vi "h.ACQ.StreamSpectraAllChannels.vi"(6 "power scales and offsets":i32[][](array[numeric]), 8 "error in":errorcluster, 11 "Connection ID":refnum<k5>) -> (0 "error out":errorcluster, 2 "Spectral Data":T1 {"Spectrum"."Spectrum, db" format="%_8g"}, 3 "Connection ID out":refnum<k5>)   [LabVIEW 2016, in "h.Library.lvlib"]
uses:
  h.Library.lvlib
  COMM/CTL/h.COMM.Command Status Enum.ctl
  COMM/CTL/h.COMM.RequestCommandOptions.ctl
  CTL/h.ACQ.SpectralData.ctl
  CTL/h.ACQ.Spectrum.ctl
panel:
  out "Message Length":u16
  out "Request Option Echo":T3=enum."Suppress Message"
  out "Message":string
  out "Content":u8[](array[numeric])
  out "Content Length":u32
  out "Status":T4
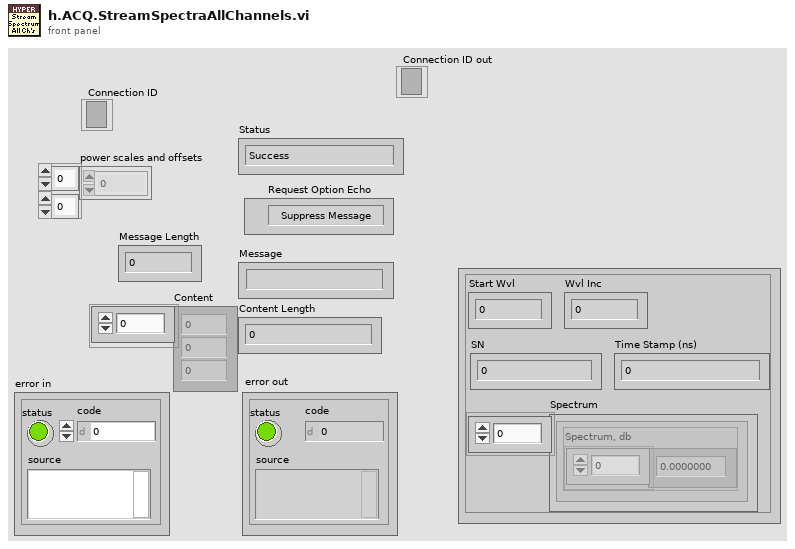
[diagram p1: front panel]
types:
  T1 = typedef "h.Library.lvlib/h.ACQ.SpectralData.ctl" = cluster{"Spectrum":T2[], "Start Wvl":dbl, "Wvl Inc":dbl, "SN":u64, "Time Stamp (ns)":u64}
  T2 = typedef "h.Library.lvlib/h.ACQ.Spectrum.ctl" = cluster{"Spectrum, db":dbl[]}
  T3 = typedef "h.Library.lvlib/h.COMM.RequestCommandOptions.ctl" = enum8{"None", "Suppress Message", "Suppress Content", "Compress"}
  T4 = typedef "h.Library.lvlib/h.COMM.Command Status Enum.ctl" = enum8{"Success", "Failed", "Error", "AccessDenied", "InvalidCommand", "InvalidNumberArguments", "InvalidArgument", ""}
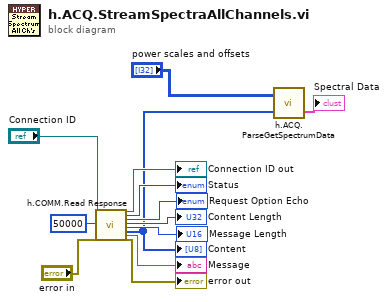
[diagram p0: block diagram]
diagram:
  n1 = call "h.COMM.Read Response.vi"("Connection ID"="Connection ID", "Timeout"=50000, "error in"="error in") -> ("Connection ID"=→"Connection ID out":refnum<k5>, "Status"=→"Status":T4, "Request Option Echo"=→"Request Option Echo":T3, "Content Length"=→"Content Length":u32, "Message Length"=→"Message Length":u16, "Content"=w5:u8[], "Message"=→"Message":string, "error out"=→"error out":errorcluster)  [unwired: 17 in]
  "Content" <- w5
  n2 = call "h.ACQ.ParseGetSpectrumData.vi"("Data from #GetSpectrum"=w5, "power scales and offsets"="power scales and offsets") -> ("Spectral Data"=→"Spectral Data":T1)  [unwired: 1 in]
